vi "BME_DG_SetDG_with_FileParameters.vi"(8 "error in (no error)":errorcluster, 10 "State":T1, 11 "DG_Number":i32) -> (0 "error out":errorcluster, 3 "return code":i32)   [LabVIEW 2009]
uses:
  Typedefs For ReadParameters()/BME_DG_BME_State.ctl
  Typedefs For ReadParameters()/BME_DG_DelayChannelData.ctl
  BME DLL/DelayGenerator.dll
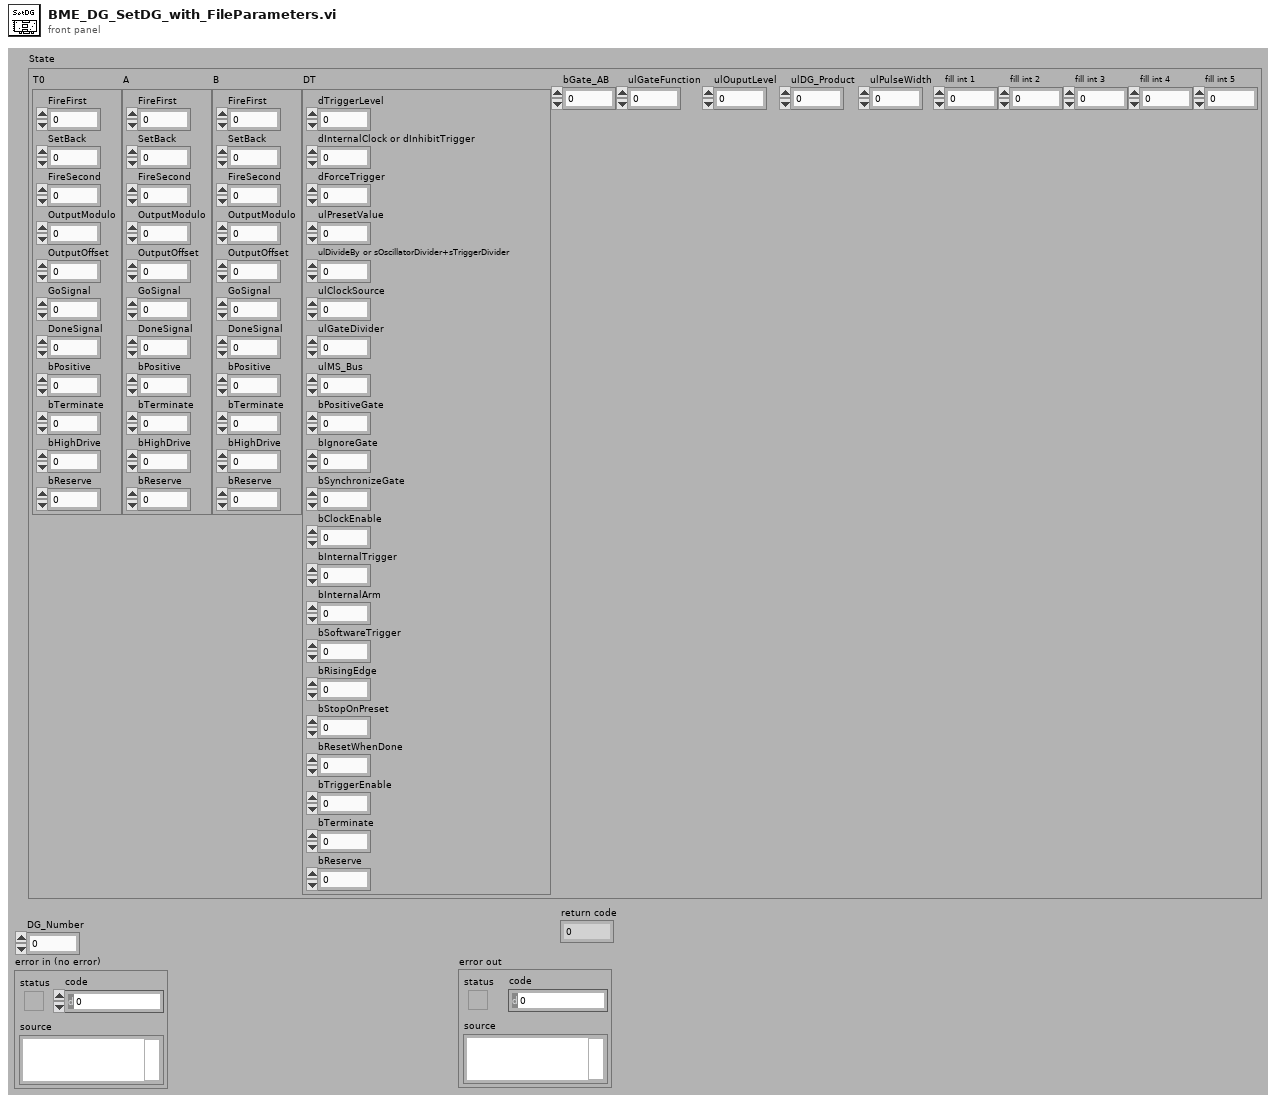
[diagram p1: front panel]
types:
  T1 = typedef "BME_DG_BME_State.ctl" = cluster{"T0":T2, "A":T2, "B":T2, "DT":cluster{"dTriggerLevel":dbl, "dInternalClock or dInhibitTrigger":dbl, "dForceTrigger":dbl, "ulPresetValue":u32, "ulDivideBy or sOscillatorDivider+sTriggerDivider":u32, "ulClockSource":u32, "ulGateDivider":u32, "ulMS_Bus":u32, "bPositiveGate":u32, "bIgnoreGate":u32, "bSynchronizeGate":u32, "bClockEnable":u32, "bInternalTrigger":u32, "bInternalArm":u32, "bSoftwareTrigger":u32, "bRisingEdge":u32, "bStopOnPreset":u32, "bResetWhenDone":u32, "bTriggerEnable":u32, "bTerminate":u32, "bReserve":u32}, "bGate_AB":u32, "ulGateFunction":u32, "ulOuputLevel":u32, "ulDG_Product":u32, "ulPulseWidth":u32, "fill int 1":i32, "fill int 2":i32, "fill int 3":i32, "fill int 4":i32, "fill int 5":i32}
  T2 = typedef "BME_DG_DelayChannelData.ctl" = cluster{"FireFirst":dbl, "SetBack":dbl, "FireSecond":dbl, "OutputModulo":u32, "OutputOffset":u32, "GoSignal":u32, "DoneSignal":u32, "bPositive":u32, "bTerminate":u32, "bHighDrive":u32, "bReserve":u32}
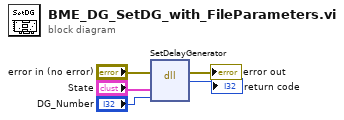
[diagram p0: block diagram]
diagram:
  n1 = dll-call lib="C:/Dokumente und Einstellungen/A2.5/Desktop/POLARIS BME DG/BME DLL/DelayGenerator.dll" fn="SetDelayGenerator"(error in="error in (no error)", "DGS"="State", "DG_Nr"="DG_Number") -> (error out=→"error out":errorcluster, "return code"=→"return code":i32)  [unwired: 4 in, 1 out]
